vi "startTcpServerA.vi"(8 "error in (no error)":errorcluster, 11 "TcpServer.lvclass":refnum<class "TcpServer.lvclass">) -> (0 "error out":errorcluster, 2 "TcpServer out":refnum<class "TcpServer.lvclass">, 3 "UserEvents":T1)   [LabVIEW 2018]
doc: "Start the TCP server A."
uses:
  src/TcpServer/TcpServer.lvclass
  src/TcpServerBase/typedef/connStatusCluster.ctl
  src/TcpServerBase/TcpServerBase.lvclass
  src/TcpServer/runServer.vi
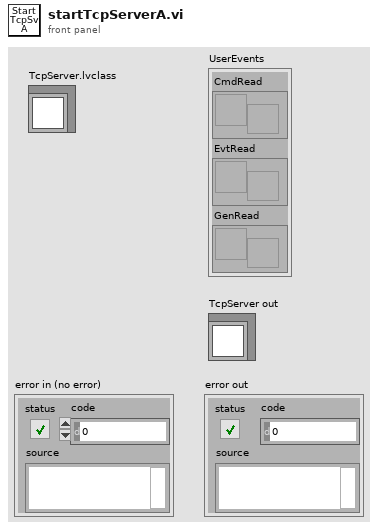
[diagram p1: front panel]
types:
  T1 = cluster{"CmdRead":refnum<user-event>, "EvtRead":refnum<user-event>, "GenRead":refnum<user-event>}
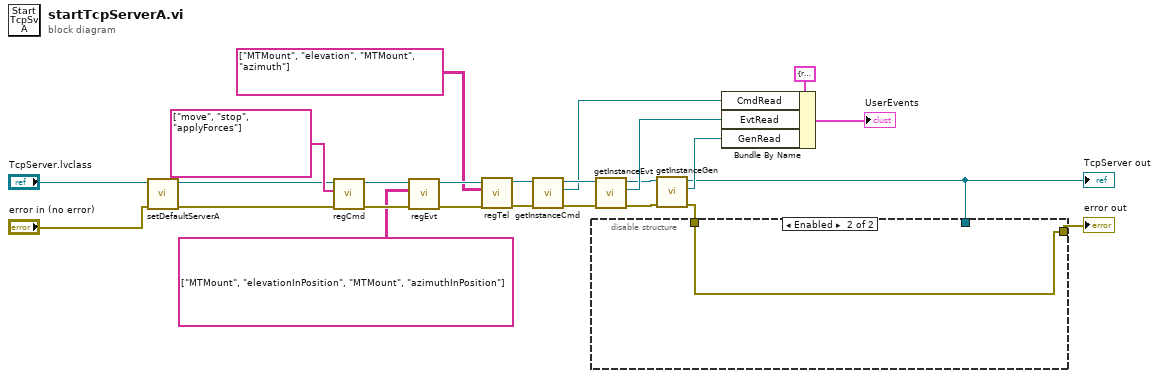
[diagram p0: block diagram]
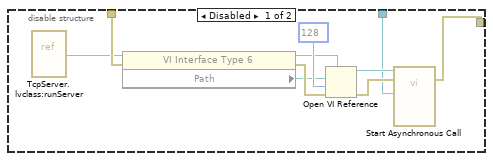
[diagram p2: hidden frame]
diagram:
  n1 = call "setDefaultServerA.vi"("error in (no error)"="error in (no error)", "TcpServer.lvclass"="TcpServer.lvclass") -> ("error out"=w5:errorcluster, "tcpServer out"=w6:refnum<class "TcpServer.lvclass">)  [unwired: 8 in]
  n2 = call "regCmd.vi"("error in (no error)"=w5, "cmdReg"=string[] ["move", "stop", "applyForces"], "tcpServer in"=w6) -> ("error out"=w21:errorcluster, "tcpServer out"=w22:refnum<class "TcpServer.lvclass">)  [unwired: 7 in]
  n3 = call "regEvt.vi"("error in (no error)"=w21, "evtReg"=string[][] [["MTMount", "elevationInPosition"], ["MTMount", "azimuthInPosition"]], "tcpServer in"=w22) -> ("error out"=w18:errorcluster, "tcpServer out"=w19:refnum<class "TcpServer.lvclass">)  [unwired: 7 in]
  n4 = call "regTel.vi"("error in (no error)"=w18, "telReg"=string[][] [["MTMount", "elevation"], ["MTMount", "azimuth"]] ("regTel"), "tcpServer in"=w19) -> ("error out"=w15:errorcluster, "tcpServer out"=w16:refnum<class "TcpServer.lvclass">)  [unwired: 7 in]
  n5 = call "getInstanceCmd.vi"("error in (no error)"=w15, "tcpServer in"=w16) -> ("error out"=w13:errorcluster, "CmdRead"=w12:refnum<user-event>, "tcpServer out"=w14:refnum<class "TcpServer.lvclass">)  [unwired: 7 in]
  n6 = call "getInstanceEvt.vi"("error in (no error)"=w13, "tcpServer in"=w14) -> ("error out"=w9:errorcluster, "EvtRead"=w11:refnum<user-event>, "tcpServer out"=w10:refnum<class "TcpServer.lvclass">)  [unwired: 7 in]
  n7 = call "getInstanceGen.vi"("error in (no error)"=w9, "tcpServer in"=w10) -> ("error out"=w3:errorcluster, "GenRead"=w8:refnum<user-event>, "tcpServer out"=w2:refnum<class "TcpServer.lvclass">)  [unwired: 7 in]
  "TcpServer out" <- w2
  n8 = disable-structure shown="Enabled" {
    disable-tunnel: w3 -> [w29 w36]
    disable-tunnel: w2 -> [w28 _]
    disable-tunnel: [w27 w36] -> w1
    frame Disabled {
      n9 = vi-ref "TcpServer.lvclass:runServer.vi"() -> (w26:refnum<vi>)
      n10 = property class="VI Interface Type 6"(reference=w26, error in=w29) -> (reference out=w31:refnum<vi>, error out=w34:errorcluster, "Path"=w30:path)
      n11 = Open VI Reference(type specifier VI Refnum (for type only)=w31, vi path=w30, options=128, error in (no error)=w34) -> (vi reference=w33:refnum<vi>, error out=w35:errorcluster)  [unwired: 2 in]
      n12 = call-by-ref "Start Asynchronous Call"(reference=w33, error in=w35, "TcpServer in"=w28) -> (error out=w27:errorcluster)  [unwired: 9 in, 3 out]
    }
    frame Enabled {
    }
  }
  "error out" <- w1
  n13 = Bundle By Name(cluster=T1 {"CmdRead"=refnum, "EvtRead"=refnum, "GenRead"=refnum}, "CmdRead"=w12, "EvtRead"=w11, "GenRead"=w8) -> (→"UserEvents":T1)
